vi "Close.vi"(8 "error in (no error)":errorcluster, 11 "VISA resource name":refnum<visa-resource-name>) -> (0 "error out":errorcluster)   [LabVIEW 2017, in "Agilent 4194.lvlib"]
doc: "This function performs the following operations:\nviClose (instrSession) and viClose (rmSession).\n\nNotes:\n\n(1) The instrument must be reinitialized to use it again."
uses:
  Agilent 4194.lvlib
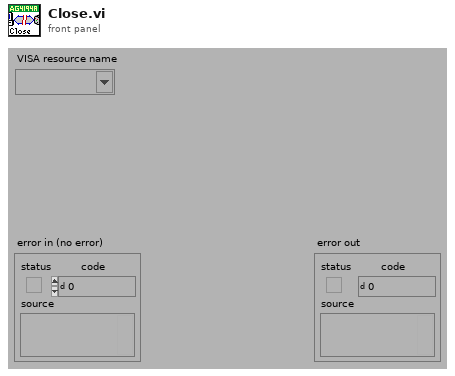
[diagram p1: front panel]
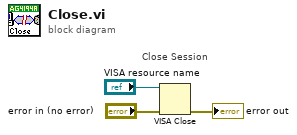
[diagram p0: block diagram]
diagram:
  # "Close Session"
  n1 = VISA Close(VISA resource name="VISA resource name", error in (no error)="error in (no error)") -> (error out=→"error out":errorcluster)
